vi "Do.vi"(8 "error in (no error)":errorcluster, 10 "Actor in":refnum<class "Actor.lvclass">, 11 "Binario Msg":refnum<class "Binario Msg.lvclass">) -> (0 "error out":errorcluster, 2 "Actor out":refnum<class "Actor.lvclass">)   [LabVIEW 2020, in "Binary.lvlib" / "Binario Msg.lvclass"]
doc: "This VI delivers the message to the actor by calling the appropriate method(s) on the actor."
uses:
  Binario Msg.lvclass
  <vilib>/ActorFramework/Actor/Actor.lvclass
  Binario Msg.lvclass/Binario Msg.ctl
  Binary/Binary.lvclass
  C:/Program Files/National Instruments/LabVIEW 2020/vi.lib/ActorFramework/Actor/Actor.lvclass
  9ef47adc-f318-494c-9b8b-6df3216d6863.vi
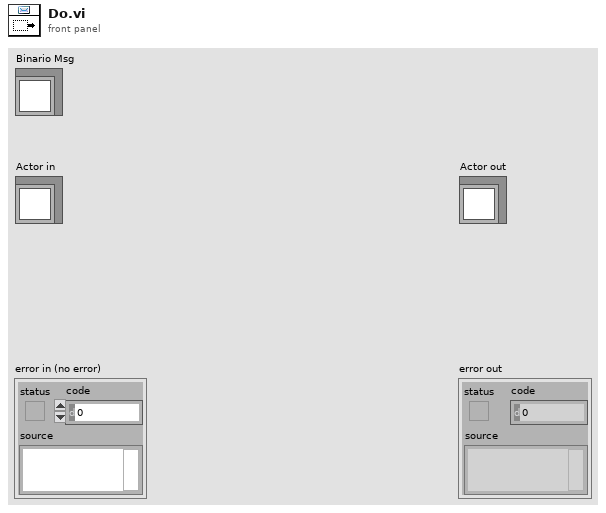
[diagram p1: front panel]
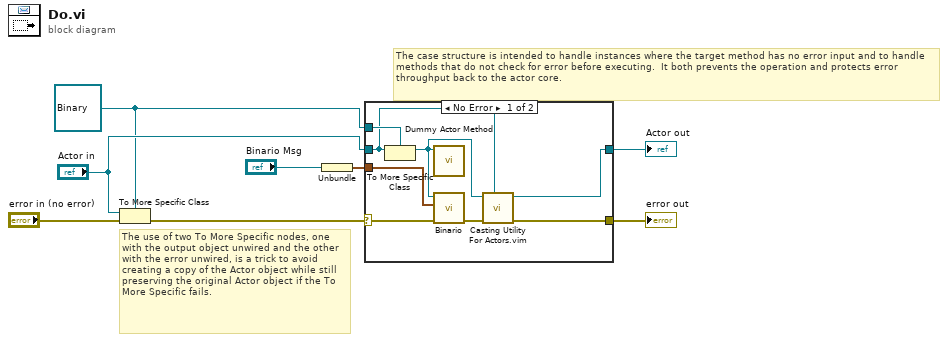
[diagram p0: block diagram]
diagram:
  w2 = refnum<class "Binary.lvclass"> refnum ("Actor in")
  # "The use of two To More Specific nodes, one with the output object unwired and the other with the error unwired, is a trick to avoid creating a copy of the Actor object while still preserving the original Actor object if the To More Specific fails."
  # "The case structure is intended to handle instances where the target method has no error input and to handle methods that do not check for error before executing.  It both prevents the operation and protects error throughput back to the actor core."
  n1 = To More Specific Class(target class=w2, reference="Actor in", error in="error in (no error)") -> (error out=w6:errorcluster)  [unwired: 1 out]
  n2 = Unbundle("Binario Msg") -> (w1:waveform(dbl))
  n3 = case shown="No Error" w6 {
    selector: w6 -> [w16 w18]
    tunnel: [w11 w18] -> w5
    tunnel: [w12 w17] -> w4
    tunnel: "Actor in" -> [w13 w17]
    tunnel: w2 -> [w14 _]
    tunnel: w1 -> [w9 _]
    frame No Error {
      n4 = To More Specific Class(target class=w14, reference=w13) -> (specific class reference=w15:refnum<class "Binary.lvclass">)  [unwired: 1 in, 1 out]
      n5 = call <resource>:"Dummy Actor Method.vi"("Actor in"=w15) -> ()  [unwired: 9 in, 2 out]
      n6 = call-dynamic "Binario.vi"("error in (no error)"=w16, "signal out"=w9, "Binary in"=w15) -> ("error out"=w10:errorcluster)  [unwired: 7 in, 1 out]
      n7 = call "Casting Utility For Actors.vim"("type"=w13, "error in (no error)"=w10, "Actor in"=w15) -> ("error out"=w11:errorcluster, "Actor out"=w12:refnum<class "Actor.lvclass">)  [unwired: 7 in]
    }
    frame Error {
      # "If type check fails, pass the original object out again."
    }
  }
  "error out" <- w5
  "Actor out" <- w4
